vi "斯坦道XML解析.vi"(11 "参数簇":T1 {"启动参数" items=["总磷"=131, "总氮"=76, "总磷海水"=147, "总氮海水"=92]}) -> (2 "步骤时间":string[](array[string]), 3 "步骤名":string[](array[string]))   [LabVIEW 2016]
uses:
  <vilib>/Utility/sysdir.llb/System Directory Type.ctl
  <vilib>/xml/Load XML File.vi
  <vilib>/xml/Close Reference(Node).vi
  <resource>/objmgr/DOMUserDefRef.rc
  <vilib>/xml/NI_XML.lvlib
panel:
  out "添加的路径":path
  out "XML字符串":string="<?xml version=\"1.0\" encoding=\"ISO-8859-1\"?>\n<bookstore>\n<book ISBN=\"978-0545128285\">\n  <title lang=\"en\">The Tales of Beedle the Bard</title>\n  <author>J. K. Rowling</author>\n  <year>2008</year>\n  <price>12.99</price>\n</book>\n<book ISBN=\"978-0316160209\">\n  <title lang=\"en\">Eclipse</title>\n  <author>Stephenie Meyer</author>\n  <year>2007</year>\n  <price>19.99</price>\n</book>\n<book ISBN=\"978-0316067928\">\n  <title lang=\"en\">Breaking Dawn</title>\n  <author>Stephenie Meyer</author>\n  <year>2008</year>\n  <price>22.99</price>\n</book>\n<book ISBN=\"978-0316017923\">\n  <title lang=\"en\">Outliers: The Story of Success</title>\n  <author>Malcolm Gladwell</author>\n  <year>2008</year>\n  <price>27.99</price>\n</book>\n<book ISBN=\"978-0596007645\">\n  <title lang=\"en\">XML in a Nutshell</title>\n  <author>Elliotte Rusty Harold</author>\n  <author>W. Scott Means</author>\n  <year>2004</year>\n  <price>39.95</price>\n</book>\n</bookstore>"
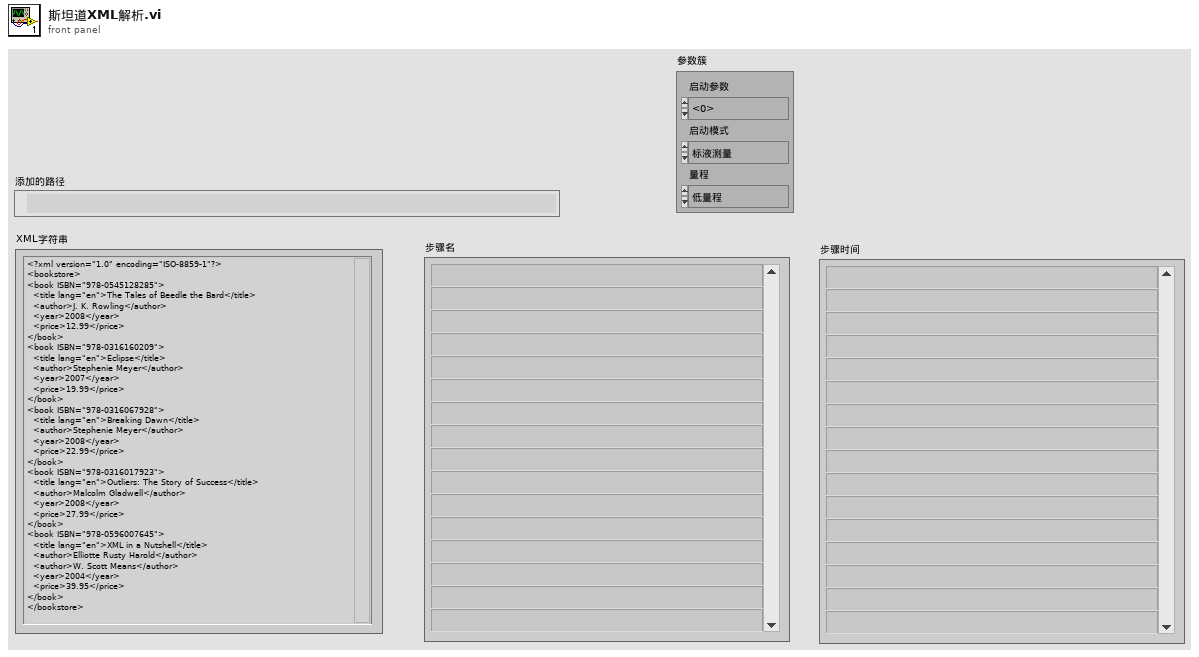
[diagram p1: front panel]
types:
  T1 = cluster{"启动模式":enum16{"标液测量", "水样测量", "零液测量", "盲样测量", "加标回收"}, "启动参数":u16, "量程":enum16{"低量程", "高量程"}}
  T2 = typedef "System Directory Type.ctl" = i32
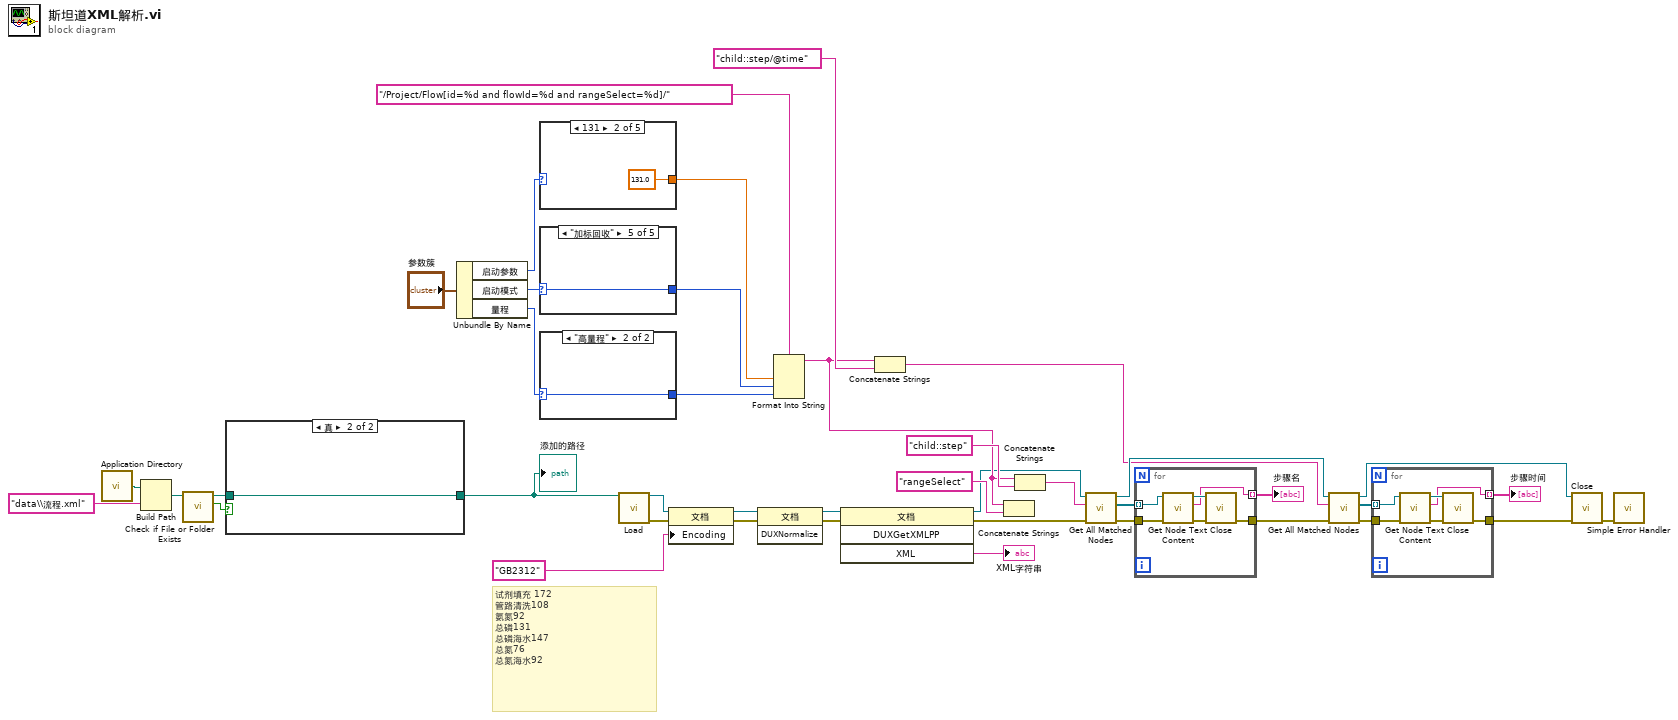
[diagram p0: block diagram]
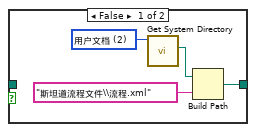
[diagram p2: hidden frame]
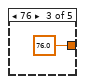
[diagram p9: hidden frame]
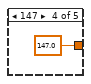
[diagram p10: hidden frame]
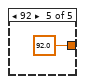
[diagram p11: hidden frame]
diagram:
  # "试剂填充 172 \n管路清洗108\n氨氮92\n总磷131\n总磷海水147\n总氮76\n总氮海水92"
  n1 = call <vilib>:"Application Directory.vi"() -> ("Application Directory"=w6:path)
  n2 = Build Path(base path=w6, name or relative path="data\\流程.xml" ("名称或相对路径")) -> (appended path=w4:path)
  n3 = call <vilib>:"Check if File or Folder Exists.vi"("path"=w4) -> ("file or folder exists?"=w3:bool, "dup path"=w2:path)  [unwired: 8 in, 1 out]
  n4 = case shown="真" w3 {
    tunnel: [w45 w46] -> w1
    tunnel: w2 -> [_ w46]
    frame False {
      w44 = T2 2 items=["用户目录"=0, "用户桌面"=1, "用户文档"=2, "用户应用程序数据"=3, "用户设置"=4, "用户临时目录"=5, "公共文档"=6, "公共应用程序数据"=7, "公共设置"=8, "公共缓存"=13, "系统核心库"=9, "系统安装库"=10, "应用程序文件"=11, "启动盘根目录"=12] ("system directory type")
      n5 = call <vilib>:"Get System Directory.vi"("system directory type"=w44) -> ("system directory"=w43:path)  [unwired: 10 in]
      n6 = Build Path(base path=w43, name or relative path="斯坦道流程文件\\流程.xml" ("名称或相对路径")) -> (appended path=w45:path)
    }
    frame True {
    }
  }
  "添加的路径" <- w1
  n7 = Unbundle By Name("参数簇") -> ("启动参数"=w9:u16, "启动模式"=w8:enum16{"标液测量", "水样测量", "零液测量", "盲样测量", "加标回收"}, "量程"=w7:enum16{"低量程", "高量程"})
  n8 = case shown="131" w9 {
    selector: w9 -> [w47 _ _ _ _]
    tunnel: [w47 131.0 ("输入 1") 76.0 ("输入 1") 147.0 ("输入 1") 92.0 ("输入 1")] -> w30
    frame Default {
    }
    frame 131 {
    }
    frame 76 {
    }
    frame 147 {
    }
    frame 92 {
    }
  }
  n9 = case shown="\"加标回收\"" w8 {
    selector: w8 -> [w52 w53 w54 w55 w56]
    tunnel: [w52 w53 w54 w55 w56] -> w29
    frame "标液测量", Default {
    }
    frame "水样测量" {
    }
    frame "零液测量" {
    }
    frame "盲样测量" {
    }
    frame "加标回收" {
    }
  }
  n10 = case shown="\"高量程\"" w7 {
    selector: w7 -> [w57 w58]
    tunnel: [w57 w58] -> w28
    frame "低量程", Default {
    }
    frame "高量程" {
    }
  }
  n11 = call-poly <vilib>:"Load.vi"("path to XML document"=w1) -> ("DOM document out"=w39:refnum<k20>, "error out"=w38:errorcluster)  [unwired: 12 in, 1 out]
  n12 = property on="属性节点" class="文档"(reference=w39, error in=w38, "Encoding"="GB2312" ("文档编码")) -> (reference out=w37:refnum<k20>, error out=w36:errorcluster)
  n13 = invoke on="Invoke Node" class="文档" method="DUXNormalize"(reference=w37, error in=w36) -> (reference out=w34:refnum<k20>, error out=w35:errorcluster)  [unwired: 1 in, 1 out]
  n14 = Format Into String(format string="/Project/Flow[id=%d and flowId=%d and rangeSelect=%d]/" ("XPath expression"), w30, w29, w28) -> (resulting string=w16:string)  [unwired: 2 in, 1 out]
  n15 = invoke on="Invoke Node" class="文档" method="DUXGetXMLPP"(reference=w34, error in=w35) -> (reference out=w12:refnum<k20>, error out=w13:errorcluster, "XML"=→"XML字符串":string)  [unwired: 2 in, 1 out]
  n16 = Concatenate Strings(w16, "child::step/@time" ("输入 4")) -> (w17:string)
  n17 = Concatenate Strings(w16, "rangeSelect" ("输入 4")) -> ()  [unwired: 1 out]
  n18 = Concatenate Strings(w16, "child::step" ("输入 4")) -> (w19:string)
  n19 = call <vilib>:"Get All Matched Nodes.vi"("error in (no error)"=w13, "XPath expression"=w19, "node in"=w12) -> ("error out"=w33:errorcluster, "node result array"=w32:refnum<k20>[], "node out"=w23:refnum<k20>)  [unwired: 6 in]
  n20 = for {
    tunnel: w33 -> [w64]
    tunnel: [w61] -> w27 mode=indexing
    tunnel: w32 -> [w60] mode=indexing
    tunnel: [w59] -> w22
    n21 = call <vilib>:"Get Node Text Content.vi"("error in (no error)"=w64, "node in"=w60) -> ("error out"=w62:errorcluster, "node text"=w61:string, "node out"=w63:refnum<k20>)  [unwired: 7 in]
    n22 = call-poly <vilib>:"Close.vi"("error in (no error)"=w62, "node"=w63) -> ("error out"=w59:errorcluster)  [unwired: 7 out]
  }
  "步骤名" <- w27
  n23 = call <vilib>:"Get All Matched Nodes.vi"("error in (no error)"=w22, "XPath expression"=w17, "node in"=w23) -> ("error out"=w25:errorcluster, "node result array"=w24:refnum<k20>[], "node out"=w11:refnum<k20>)  [unwired: 6 in]
  n24 = for {
    tunnel: w25 -> [w70]
    tunnel: [w67] -> w21 mode=indexing
    tunnel: w24 -> [w66] mode=indexing
    tunnel: [w65] -> w14
    n25 = call <vilib>:"Get Node Text Content.vi"("error in (no error)"=w70, "node in"=w66) -> ("error out"=w68:errorcluster, "node text"=w67:string, "node out"=w69:refnum<k20>)  [unwired: 7 in]
    n26 = call-poly <vilib>:"Close.vi"("error in (no error)"=w68, "node"=w69) -> ("error out"=w65:errorcluster)  [unwired: 7 out]
  }
  "步骤时间" <- w21
  n27 = call-poly <vilib>:"Close.vi"("error in (no error)"=w14, "node"=w11) -> ("error out"=w26:errorcluster)  [unwired: 7 out]
  n28 = call <vilib>:"Simple Error Handler.vi"("error in (no error)"=w26) -> ()  [unwired: 4 in, 5 out]
